vi "Maintain Heading.vi"(9 "PID gains":T1={"proportional gain (Kc)"=0.02, "integral time (Ti, min)"=0.025, "derivative time (Td, min)"=0.0} {"derivative time (Td, min)" format="%.3f"; "integral time (Ti, min)" format="%.3f"; "proportional gain (Kc)" format="%.3f"}, 10 "NavX Yaw":dbl=-2.8700000000000045, 11 "Raw Driver Joystick X2":dbl) -> (3 "Driver Joystick X2":dbl)   [LabVIEW 2014]
uses:
  <vilib>/Rock Robotics/WPI/DriverStation/WPI_DriverStationRobotMode2.ctl
  Begin/Global Variables.vi
  <vilib>/addons/control/pid/pid.llb/PID (DBL).vi
  <vilib>/addons/control/pid/NI_PID_pid.lvlib
panel:
  in  "Deadband":dbl=0.05 format="%#_13g"
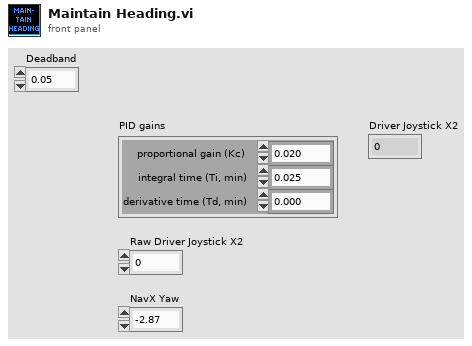
[diagram p1: front panel]
types:
  T1 = cluster{"proportional gain (Kc)":dbl, "integral time (Ti, min)":dbl, "derivative time (Td, min)":dbl}
  T2 = typedef "WPI_DriverStationRobotMode2.ctl" = enum16{"Autonomous Disabled", "Autonomous Enabled", "Teleop Disabled", "Teleop Enabled", "Disconnected", "Finish", "Test Disabled", "Test Enabled", "Emergency Stopped"}
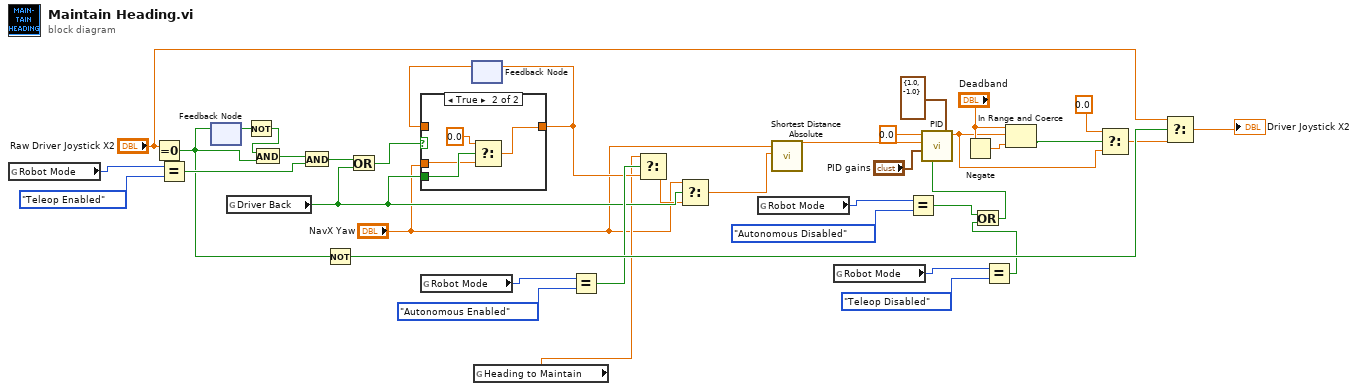
[diagram p0: block diagram]
diagram:
  n1 = global read "Global Variables.vi" "Robot Mode"() -> (w22:T2)
  n2 = Equal To 0?(x="Raw Driver Joystick X2") -> (x = 0?=w25:bool)
  n3 = Equal?(x=w22, y=WPI_DriverStationRobotMode2."Teleop Enabled") -> (x = y?=w37:bool)
  n4 = feedback #1() -> (w27:bool)  [unwired: 1 in]
  n5 = feedback-in #1(w25) -> ()
  n6 = global read "Global Variables.vi" "Driver Back"() -> (w9:bool)
  n7 = Not(x=w27) -> (.not. x?=w26:bool)
  n8 = And(x=w26, y=w25) -> (x .and. y?=w35:bool)
  n9 = And(x=w35, y=w37) -> (x .and. y?=w38:bool)
  n10 = Not(x=w25) -> (.not. x?=w24:bool)
  n11 = Or(x=w38, y=w9) -> (x .or. y?=w39:bool)
  n12 = global read "Global Variables.vi" "Robot Mode"() -> (w19:T2)
  n13 = feedback #2() -> (w23:dbl)  [unwired: 1 in]
  n14 = case shown="True" w39 {
    tunnel: w9 -> [_ w44]
    tunnel: "NavX Yaw" -> [_ w42]
    tunnel: [w40 w41] -> w10
    tunnel: w23 -> [w40 _]
    frame False {
    }
    frame True {
      n15 = Select(t=0.0, s=w44, f=w42) -> (s? t:f=w41:dbl)
    }
  }
  n16 = feedback-in #2(w10) -> ()
  n17 = global read "Global Variables.vi" "Heading to Maintain"() -> (w3:dbl)
  n18 = Equal?(x=w19, y=WPI_DriverStationRobotMode2."Autonomous Enabled") -> (x = y?=w18:bool)
  n19 = Select(t=w3, s=w18, f=w10) -> (s? t:f=w8:dbl)
  n20 = Select(t="NavX Yaw", s=w9, f=w8) -> (s? t:f=w7:dbl)
  n21 = global read "Global Variables.vi" "Robot Mode"() -> (w17:T2)
  n22 = call "Shortest Distance Absolute.vi"("current"=w7, "target"="NavX Yaw") -> ("shortest angle"=w31:dbl)  [unwired: 9 in]
  n23 = global read "Global Variables.vi" "Robot Mode"() -> (w14:T2)
  n24 = Equal?(x=w17, y=WPI_DriverStationRobotMode2."Autonomous Disabled") -> (x = y?=w13:bool)
  n25 = Negate(x="Deadband") -> (-x=w34:dbl)
  n26 = Equal?(x=w14, y=WPI_DriverStationRobotMode2."Teleop Disabled") -> (x = y?=w12:bool)
  n27 = Or(x=w13, y=w12) -> (x .or. y?=w11:bool)
  n28 = call-poly <vilib>:"PID.vi"("reinitialize? (F)"=w11, "output range"=cluster{"output high":dbl, "output low":dbl} {"output high"=1.0, "output low"=-1.0}, "PID gains"="PID gains", "process variable"=w31, "setpoint"=0.0) -> ("output"=w5:dbl)  [unwired: 5 in, 1 out]
  n29 = In Range and Coerce(upper limit="Deadband", x=w5, lower limit=w34) -> (In Range?=w6:bool)  [unwired: 1 out]
  n30 = Select(t=0.0, s=w6, f=w5) -> (s? t:f=w4:dbl)
  n31 = Select(t="Raw Driver Joystick X2", s=w24, f=w4) -> (s? t:f=→"Driver Joystick X2":dbl)
